vi "CompleteAutoTest.vi"(8 "error in (no error)":errorcluster, 11 "ExecutionControls in":refnum<class "ExecutionControls.lvclass">) -> (0 "error out":errorcluster, 3 "ExecutionControls out":refnum<class "ExecutionControls.lvclass">)   [LabVIEW 2019, in "ExecutionControls.lvclass"]
uses:
  ExecutionControls.lvclass
  <vilib>/Utility/miscctls.llb/LVForegroundBackgroundColorsTypeDef.ctl
  ExecutionControls.lvclass/ExecutionControls.ctl
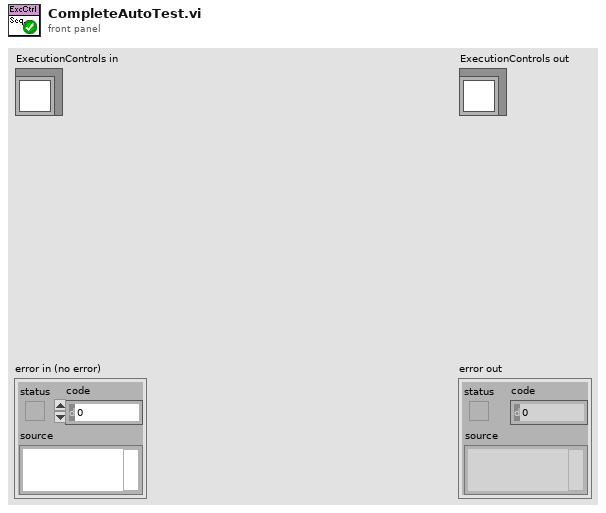
[diagram p1: front panel]
types:
  T1 = enum32{"Page Enabled", "Page Disabled", "Page Disabled & Grayed"}
  T2 = enum8{"Enabled", "Disabled", "Disabled and Grayed Out"}
  T3 = typedef "LVForegroundBackgroundColorsTypeDef.ctl" = cluster{"Foreground Color":u32, "Background Color":u32}
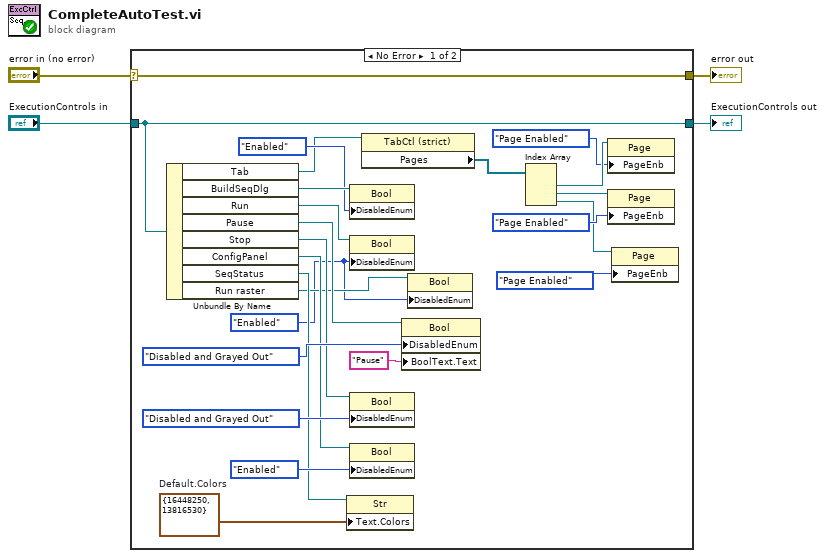
[diagram p0: block diagram]
diagram:
  n1 = case shown="No Error" "error in (no error)" {
    selector: "error in (no error)" -> [w28 w30]
    tunnel: [w28 w30] -> w2
    tunnel: [w18 w29] -> w3
    tunnel: "ExecutionControls in" -> [w18 w29]
    frame No Error {
      w10 = T3 {"Foreground Color"=16448250, "Background Color"=13816530}  # Default.Colors
      w5 = T2."Enabled" ("Disabled")
      n2 = Unbundle By Name(w18) -> ("Tab"=w17:refnum<vi>, "BuildSeqDlg"=w27:refnum<vi>, "Run"=w25:refnum<vi>, "Pause"=w21:refnum<vi>, "Stop"=w20:refnum<vi>, "ConfigPanel"=w19:refnum<vi>, "SeqStatus"=w9:refnum<vi>, "Run raster"=w6:refnum<vi>)
      n3 = property class="Str"(reference=w9, "Text.Colors"=w10) -> ()  [unwired: 1 in, 2 out]
      n4 = property class="Bool"(reference=w27, "DisabledEnum"=T2."Enabled" ("Disabled")) -> ()  [unwired: 1 in, 2 out]
      n5 = property class="Bool"(reference=w25, "DisabledEnum"=w5) -> ()  [unwired: 1 in, 2 out]
      n6 = property class="Bool"(reference=w20, "DisabledEnum"=T2."Disabled and Grayed Out" ("Disabled")) -> ()  [unwired: 1 in, 2 out]
      n7 = property class="Bool"(reference=w19, "DisabledEnum"=T2."Enabled" ("Disabled")) -> ()  [unwired: 1 in, 2 out]
      n8 = property class="TabCtl (strict)"(reference=w17) -> ("Pages"=w16:refnum<vi>[])  [unwired: 1 in, 2 out]
      n9 = property class="Bool"(reference=w21, "DisabledEnum"=T2."Disabled and Grayed Out" ("Disabled"), "BoolText.Text"="Pause" ("Boolean Text.Text")) -> ()  [unwired: 1 in, 2 out]
      n10 = property class="Bool"(reference=w6, "DisabledEnum"=w5) -> ()  [unwired: 1 in, 2 out]
      n11 = Index Array(array=w16) -> (element #1=w14:refnum<vi>, element #2=w15:refnum<vi>, element #3=w8:refnum<vi>)  [unwired: 3 in]
      n12 = property class="Page"(reference=w14, "PageEnb"=T1."Page Enabled" ("Page Enabled State")) -> ()  [unwired: 1 in, 2 out]
      n13 = property class="Page"(reference=w15, "PageEnb"=T1."Page Enabled" ("Page Enabled State")) -> ()  [unwired: 1 in, 2 out]
      n14 = property class="Page"(reference=w8, "PageEnb"=T1."Page Enabled" ("Page Enabled State")) -> ()  [unwired: 1 in, 2 out]
    }
    frame Error {
    }
  }
  "error out" <- w2
  "ExecutionControls out" <- w3
